vi "Set Output Voltage.vi"(8 "error in (no error)":errorcluster, 10 "Voltage [V]":dbl, 11 "Mock Voltage Output In":refnum<class "Mock Voltage Output.lvclass">) -> (0 "error out":errorcluster, 3 "Mock Voltage Output Out":refnum<class "Mock Voltage Output.lvclass">)   [LabVIEW 2020, in "High Level PSU With Tests.lvlib" / "Mock Voltage Output.lvclass"]
uses:
  Mock Voltage Output.lvclass
  Mock Voltage Output.lvclass/Mock Voltage Output.ctl
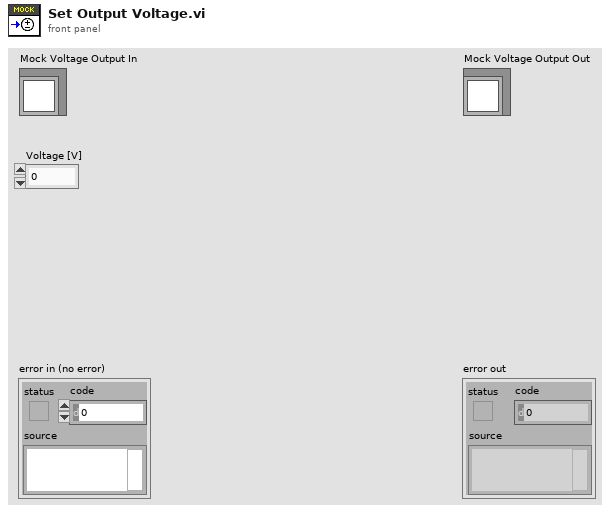
[diagram p1: front panel]
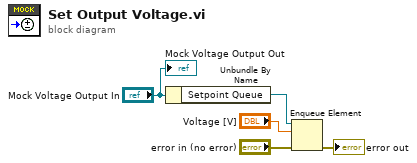
[diagram p0: block diagram]
diagram:
  n1 = Unbundle By Name("Mock Voltage Output In") -> ("Setpoint Queue"=w4:refnum<queue>)
  n2 = Enqueue Element(queue=w4, element="Voltage [V]", error in (no error)="error in (no error)") -> (error out=→"error out":errorcluster)  [unwired: 1 in, 2 out]
  "Mock Voltage Output Out" <- "Mock Voltage Output In"
